vi "GT Read Watch.vi"(6 "pReadCount":u32, 7 "bufferSize":u32, 8 "error in (no error)":errorcluster caption="错误输入（无错误）", 9 "pBuffer":dbl[](array[numeric]), 10 "varIndex":i16, 11 "cardNum":i16) -> (0 "error out":errorcluster caption="错误输出", 1 "pBuffer out":dbl[](array[numeric]), 3 "function return":i16, 4 "pReadCount out":u32)   [LabVIEW 2020, in "gts1.lvlib"]
doc: "GT_API GT_ReadWatch(short cardNum,short varIndex,double *pBuffer,unsigned long bufferSize,unsigned long *pReadCount);"
uses:
  gts1.lvlib
  dll/32bit/multi_card/gts.dll
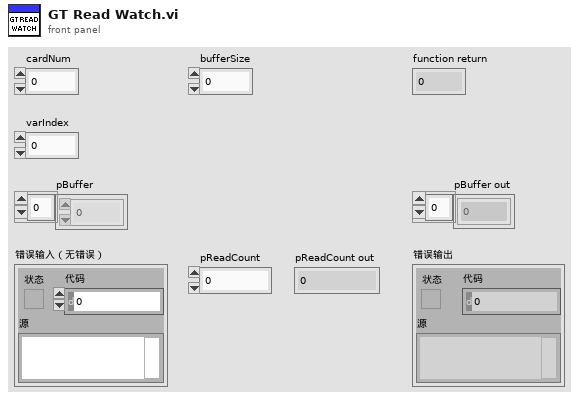
[diagram p1: front panel]
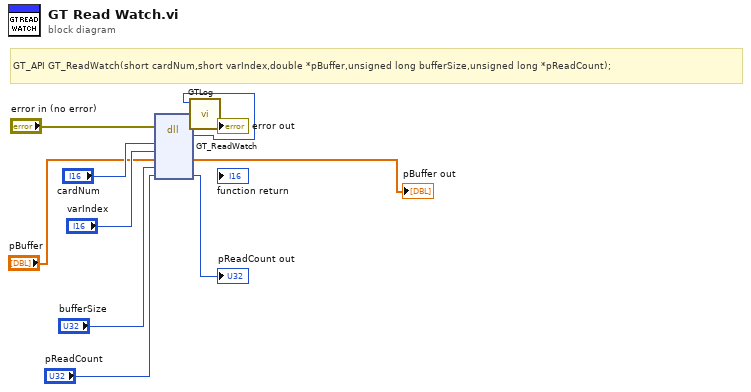
[diagram p0: block diagram]
diagram:
  # "GT_API GT_ReadWatch(short cardNum,short varIndex,double *pBuffer,unsigned long bufferSize,unsigned long *pReadCount);"
  n1 = dll-call lib="C:/1228/dll/32bit/multi_card/gts.dll" fn="GT_ReadWatch"(error in="error in (no error)", "cardNum"="cardNum", "varIndex"="varIndex", "pBuffer"="pBuffer", "bufferSize"="bufferSize", "pReadCount"="pReadCount") -> (error out=w5:errorcluster, "返回类型"=w1:i16, "pBuffer"=→"pBuffer out":dbl[], "pReadCount"=→"pReadCount out":u32)  [unwired: 5 in, 1 out]
  n2 = call "GTLog.vi"("error in (no error)"=w5, "Numeric"=w1) -> ("error out"=→"error out":errorcluster)  [unwired: 9 in]
